vi "Main.vi"() -> ()   [LabVIEW 2015]
uses:
  State.ctl
  Power Meter/Parent/Power Meter.lvclass
  Temperature Device/Parent/Temperature Device.lvclass
  Global Data.ctl
  Data.ctl
  Power Meter/Parent/Power Data.ctl
  <vilib>/Utility/config.llb/Read Key (I32).vi
  <vilib>/Utility/config.llb/Read Key (Double).vi
  <vilib>/Utility/config.llb/Read Key (String).vi
  <vilib>/Utility/config.llb/NI_LVConfig.lvlib
panel:
  out "Channel 3":dbl(graph)
  in  "Simulate":bool
  out "GPIB Error":errorcluster
  out "current time":timestamp format="%<%H:%M:%S%2u>T"
  out "Temperature":cluster{"Data[0]":dbl, "Data[1]":dbl}(graph)
  in  "disp":T1(ring) caption="Display Variable"
  out "Channel 2":dbl(graph)
  out "Channel 1":dbl(graph)
  in  "texe":i32=100
  in  "twait":dbl=1.0
  # "Actual"
  # "Simulated"
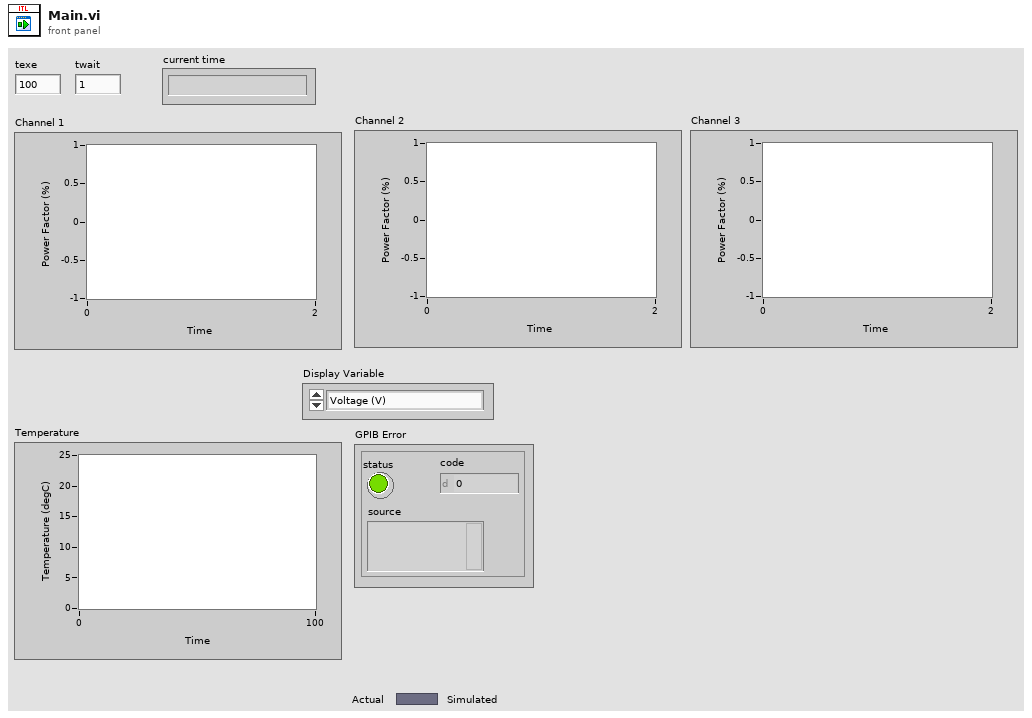
[diagram p1: front panel]
types:
  T1 = enum16{"Voltage (V)", "Amperage (A)", "Power (W)", "Power Factor (%)", "Total Voltage Distortion (%)", "Total Amperage Distortion (%)"}
  T2 = typedef "State.ctl" = enum16{"Configure", "Collect Data", "Wait", "Stop"}
  T3 = typedef "Global Data.ctl" = cluster{"Power Data":T4[], "Time":timestamp, "Temperature":dbl[]}
  T4 = typedef "Data.ctl" = cluster{"Voltage":dbl, "Amperage":dbl, "Wattage":dbl, "Power Factor":dbl, "Voltage Distortion":dbl, "Amperage Distortion":dbl}
  T5 = typedef "Power Meter.lvclass/Power Data.ctl" = cluster{"V":dbl, "I":dbl, "P":dbl, "PF":dbl, "VTHD":dbl, "ITHD":dbl}
  T6 = typedef "NI_LVConfig.lvlib/Config Data RefNum.ctl" = refnum<k1>
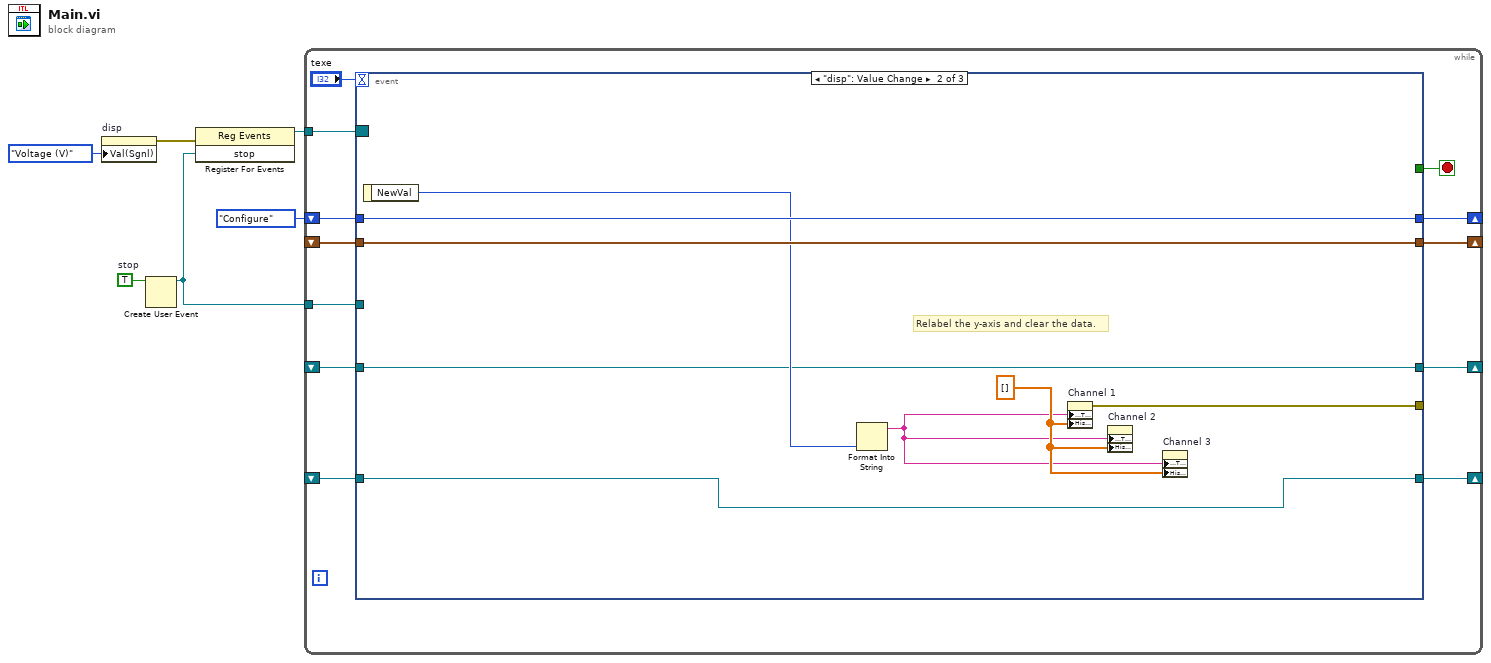
[diagram p0: block diagram]
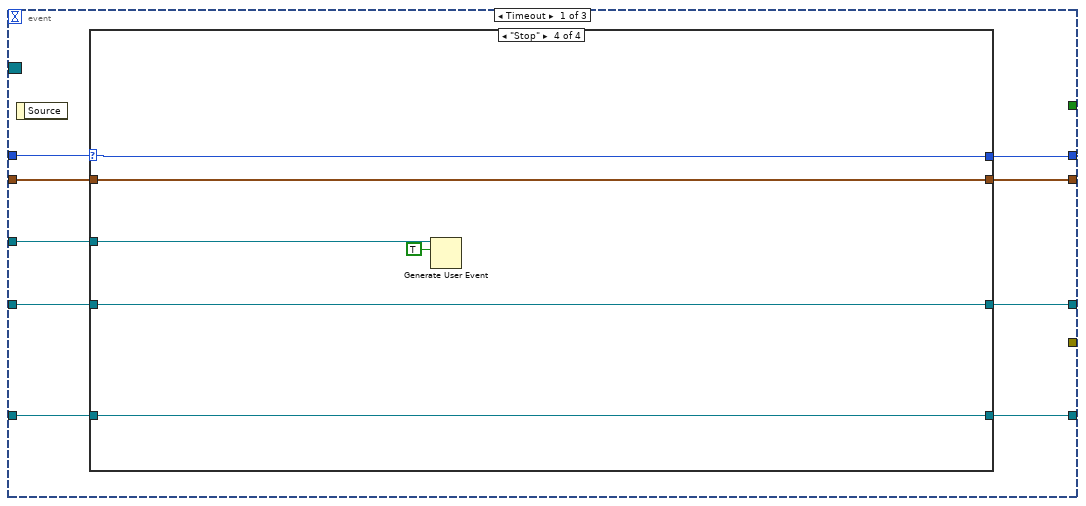
[diagram p2: hidden frame]
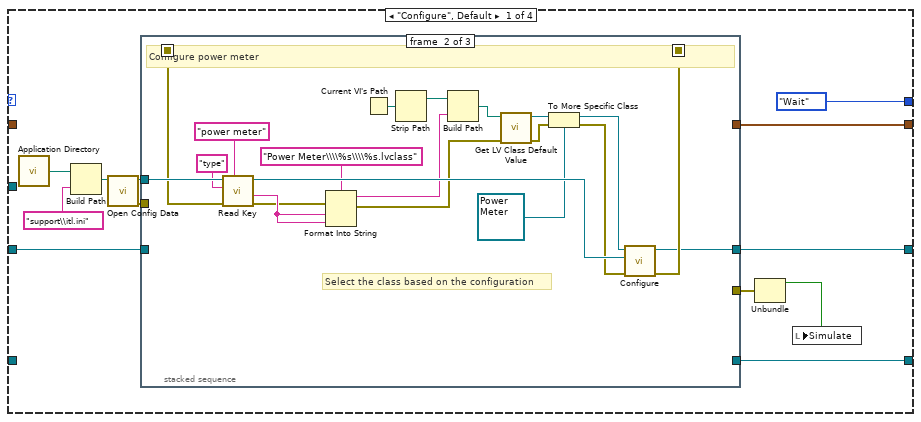
[diagram p3: hidden frame]
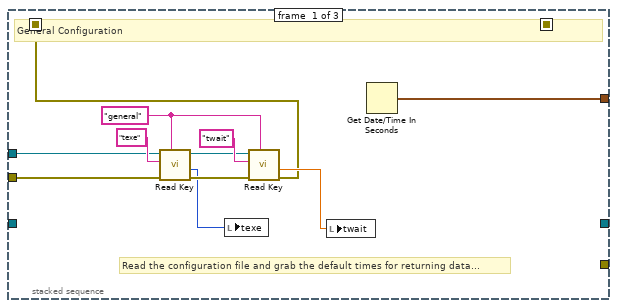
[diagram p4: hidden frame]
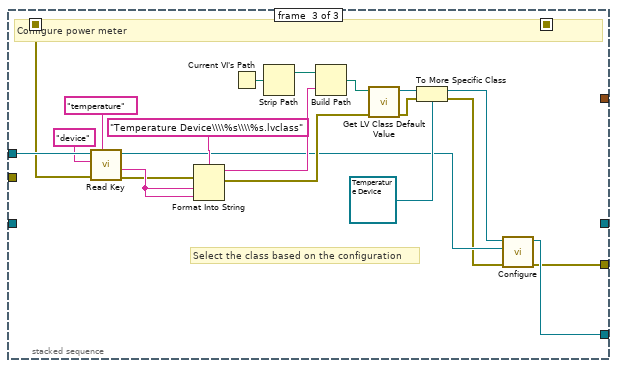
[diagram p5: hidden frame]
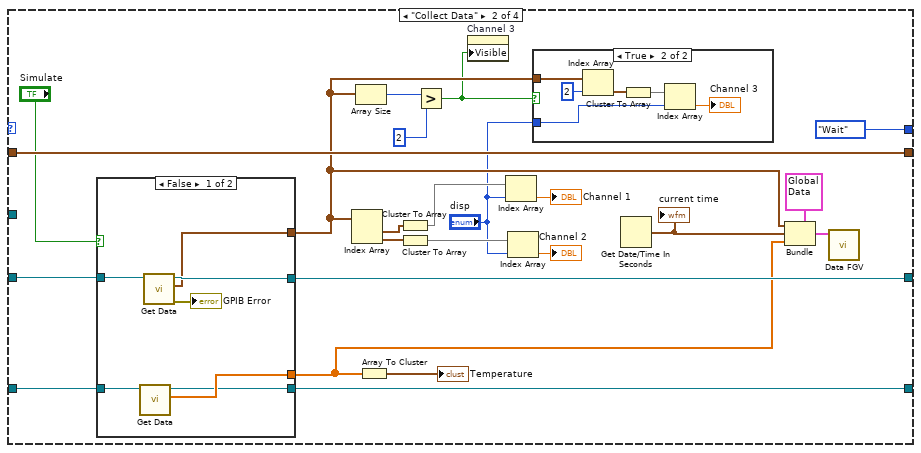
[diagram p6: hidden frame]
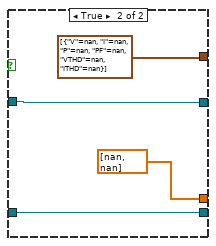
[diagram p8: hidden frame]
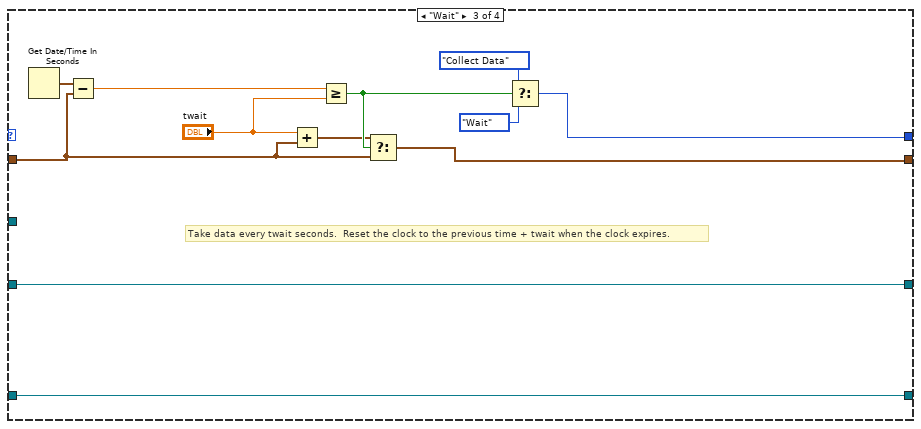
[diagram p9: hidden frame]
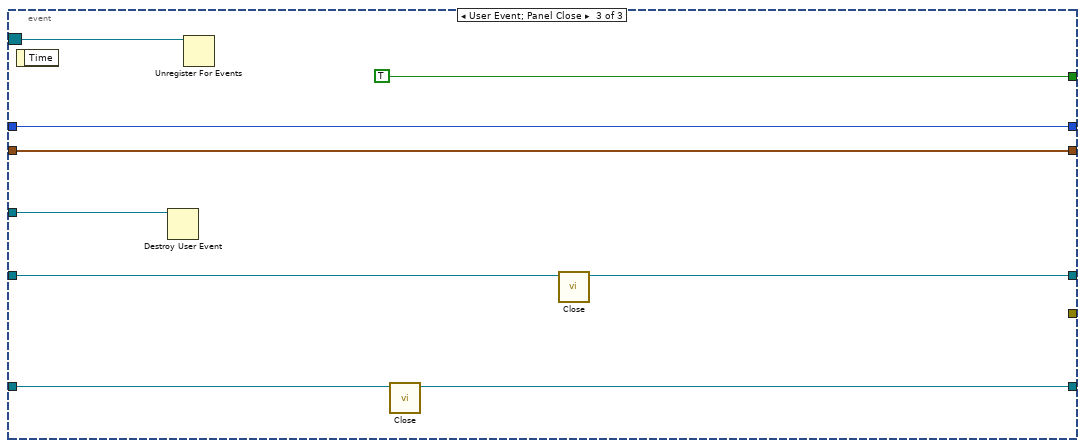
[diagram p10: hidden frame]
diagram:
  w5 = TRUE  # stop
  n1 = property on="disp" class="Enum (strict)"("Val(Sgnl)"=T1."Voltage (V)" ("Value (Signaling)")) -> (error out=w1:errorcluster)  [unwired: 2 in, 1 out]
  n2 = Create User Event(user event datatype=w5) -> (user event=w3:refnum<user-event>)  [unwired: 1 in, 1 out]
  n3 = register-events(error in=w1, w3) -> (reference out=w4:refnum<event-registration>)  [unwired: 1 in, 1 out]
  n4 = while {
    shift-right: [w14] -> _
    shift-left: _ -> [w16]
    shift-right: [w17] -> _
    shift-left: State."Configure" -> [w18]
    tunnel: w4 -> [w13]
    tunnel: w3 -> [w12]
    shift-right: [w9] -> _
    shift-left: _ -> [w10]
    shift-right: [w8] -> _
    shift-left: _ -> [w7]
    stop <- w15 stop-if-true
    n5 = event shown="[1] \"disp\": Value Change" {
      selector: w13 -> [_ _ w161]
      dyn-events: _ -> [_ _ _]
      timeout: "texe" -> [_ _ _]
      tunnel: w18 -> [w27 w155 w163]
      tunnel: [w26 w155 w163] -> w17
      tunnel: w16 -> [w25 w156 w164]
      tunnel: [_ _ TRUE] -> w15
      tunnel: [w24 w156 w164] -> w14
      tunnel: [_ w154 _] -> _
      tunnel: w12 -> [w23 _ w162]
      tunnel: w10 -> [w22 w152 w160]
      tunnel: [w21 w152 w159] -> w9
      tunnel: [w20 w151 w157] -> w8
      tunnel: w7 -> [w19 w151 w158]
      event Timeout {
        n6 = event-data() -> ()  [unwired: 1 in, 1 out]
        n7 = case shown="\"Stop\"" w27 {
          selector: w27 -> [_ _ _ w146]
          tunnel: [State."Wait" State."Wait" w139 w146] -> w26
          tunnel: w25 -> [_ w112 w134 w145]
          tunnel: [w35 w112 w133 w145] -> w24
          tunnel: w23 -> [_ _ _ w148]
          tunnel: w22 -> [w30 w105 w132 w144]
          tunnel: [w29 w104 w132 w144] -> w21
          tunnel: [w28 w98 w131 w143] -> w20
          tunnel: w19 -> [_ w99 w131 w143]
          frame "Configure", Default {
            n8 = call <vilib>:"Application Directory.vi"() -> ("Application Directory"=w39:path)
            n9 = Build Path(base path=w39, name or relative path="support\\itl.ini") -> (appended path=w37:path)
            n10 = call <vilib>:"Open Config Data.vi"("configuration file path"=w37) -> ("error out"=w34:errorcluster, "refnum"=w36:T6)  [unwired: 8 in, 1 out]
            n11 = stacked-sequence {
              seq-local: [w41 _ _] -> [_ w54 w72]
              seq-local: [_ w70 _] -> [_ _ _]
              tunnel: w36 -> [w45 w68 w90]
              tunnel: [w42 _ _] -> w35
              tunnel: [_ _ w71] -> w33
              tunnel: w34 -> [w40 _ _]
              tunnel: w30 -> [_ _ _]
              tunnel: [_ w69 _] -> w29
              tunnel: [_ _ w73] -> w28
              frame #0 {
                w47 = "general" ("section")
                # "Read the configuration file and grab the default times for returning data..."
                # "General Configuration"
                n12 = call-poly <vilib>:"Read Key.vi"("section"=w47, "error in (no error)"=w40, "key"="texe", "refnum"=w45) -> ("error out"=w50:errorcluster, "value"=w44:i32, "refnum out"=w46:T6)  [unwired: 4 in, 1 out]
                n13 = local write "texe"(w44) -> ()
                n14 = call-poly <vilib>:"Read Key.vi"("section"=w47, "error in (no error)"=w50, "key"="twait", "refnum"=w46) -> ("error out"=w41:errorcluster, "value"=w43:dbl)  [unwired: 4 in, 2 out]
                n15 = local write "twait"(w43) -> ()
                n16 = Get Date/Time In Seconds() -> (seconds since 1Jan1904=w42:timestamp)
              }
              frame #1 {
                # "Select the class based on the configuration"
                # "Configure power meter"
                n17 = call-poly <vilib>:"Read Key.vi"("section"="power meter", "error in (no error)"=w54, "key"="type", "refnum"=w68) -> ("error out"=w53:errorcluster, "value"=w61:string, "refnum out"=w65:T6)  [unwired: 4 in, 1 out]
                n18 = Format Into String(format string="Power Meter\\\\%s\\\\%s.lvclass", error in=w53, w61, w61) -> (resulting string=w60:string, error out=w52:errorcluster)  [unwired: 1 in]
                n19 = Current VI's Path() -> (path=w64:path)
                n20 = Strip Path(path=w64) -> (stripped path=w63:path)  [unwired: 1 out]
                n21 = Build Path(base path=w63, name or relative path=w60) -> (appended path=w59:path)
                n22 = call <vilib>:"Get LV Class Default Value.vi"("error in (no error)"=w52, "class path"=w59) -> ("error out"=w58:errorcluster, "object"=w57:refnum<class>)  [unwired: 8 in]
                n23 = To More Specific Class(target class=refnum<class "Power Meter.lvclass"> refnum ("Power Meter"), reference=w57, error in=w58) -> (specific class reference=w55:refnum<class "Power Meter.lvclass">, error out=w51:errorcluster)
                n24 = call-dynamic "Configure.vi"("error in (no error)"=w51, "ConfigRef In"=w65, "Power Meter in"=w55) -> ("error out"=w70:errorcluster, "Power Meter out"=w69:refnum<class "Power Meter.lvclass">)  [unwired: 7 in]
              }
              frame #2 {
                # "Select the class based on the configuration"
                # "Configure power meter"
                n25 = call-poly <vilib>:"Read Key.vi"("section"="temperature", "error in (no error)"=w72, "key"="device", "refnum"=w90) -> ("error out"=w79:errorcluster, "value"=w84:string, "refnum out"=w75:T6)  [unwired: 4 in, 1 out]
                n26 = Format Into String(format string="Temperature Device\\\\%s\\\\%s.lvclass", error in=w79, w84, w84) -> (resulting string=w83:string, error out=w78:errorcluster)  [unwired: 1 in]
                n27 = Current VI's Path() -> (path=w87:path)
                n28 = Strip Path(path=w87) -> (stripped path=w86:path)  [unwired: 1 out]
                n29 = Build Path(base path=w86, name or relative path=w83) -> (appended path=w82:path)
                n30 = call <vilib>:"Get LV Class Default Value.vi"("error in (no error)"=w78, "class path"=w82) -> ("error out"=w81:errorcluster, "object"=w80:refnum<class>)  [unwired: 8 in]
                n31 = To More Specific Class(target class=refnum<class "Temperature Device.lvclass"> refnum ("Temperature Device"), reference=w80, error in=w81) -> (specific class reference=w76:refnum<class "Temperature Device.lvclass">, error out=w74:errorcluster)
                n32 = call-dynamic "Configure.vi"("error in (no error)"=w74, "ConfigRef In"=w75, "Temperature Device in"=w76) -> ("error out"=w71:errorcluster, "Temperature Device out"=w73:refnum<class "Temperature Device.lvclass">)  [unwired: 7 in]
              }
            }
            n33 = Unbundle(w33) -> ("status"=w32:bool)  [unwired: 2 out]
            n34 = local write "Simulate"(w32) -> ()
          }
          frame "Collect Data" {
            n35 = case shown="False" "Simulate" {
              tunnel: [w122 dbl[] [nan, nan] ("Data")] -> w97
              tunnel: w105 -> [w126 w130]
              tunnel: [w125 w130] -> w104
              tunnel: [w124 T5[] [{"V"=nan, "I"=nan, "P"=nan, "PF"=nan, "VTHD"=nan, "ITHD"=nan}] ("Data Out")] -> w93
              tunnel: w99 -> [w123 w128]
              tunnel: [w121 w128] -> w98
              frame False {
                n36 = call-dynamic "Get Data.vi"("Temperature Device in"=w123) -> ("Data"=w122:dbl[], "Temperature Device out"=w121:refnum<class "Temperature Device.lvclass">)  [unwired: 8 in, 1 out]
                n37 = call-dynamic "Get Data.vi"("Power Meter in"=w126) -> ("error out"=→"GPIB Error":errorcluster, "Data Out"=w124:T5[], "Power Meter out"=w125:refnum<class "Power Meter.lvclass">)  [unwired: 8 in]
              }
              frame True {
              }
            }
            n38 = Index Array(array=w93) -> (element #1=w103:T5, element #2=w101:T5)  [unwired: 2 in]
            n39 = Array Size(array=w93) -> (size(s)=w95:i32)
            n40 = Array To Cluster(array=w97) -> (cluster=→"Temperature":cluster{"Data[0]":dbl, "Data[1]":dbl})
            n41 = Cluster To Array(cluster=w103) -> (array=w102:dbl[])
            n42 = Cluster To Array(cluster=w101) -> (array=w100:dbl[])
            n43 = Greater?(x=w95, y=2) -> (0:w91:bool)
            n44 = property on="Channel 3" class="WFChart (strict)"("Visible"=w91) -> ()  [unwired: 2 in, 2 out]
            n45 = Index Array(array=w102, index="disp") -> (element=→"Channel 1":dbl)
            n46 = Index Array(array=w100, index="disp") -> (element=→"Channel 2":dbl)
            n47 = case shown="True" w91 {
              tunnel: w93 -> [_ w119]
              tunnel: "disp" -> [_ w115]
              frame False {
              }
              frame True {
                n48 = Index Array(array=w119, index=2) -> (element=w117:T5)
                n49 = Cluster To Array(cluster=w117) -> (array=w116:dbl[])
                n50 = Index Array(array=w116, index=w115) -> (element=→"Channel 3":dbl)
              }
            }
            n51 = Get Date/Time In Seconds() -> (seconds since 1Jan1904=w110:timestamp)
            "current time" <- w110
            n52 = Bundle(cluster=T3 {"Power Data"=[], "Time"=timestamp(0 s since 1904-01-01), "Temperature"=[]} ("Data In"), "Power Data"=w93, "Time"=w110, "Temperature"=w97) -> (w109:T3)
            n53 = call "Data FGV.vi"("Data In"=w109) -> ()  [unwired: 10 in, 1 out]
          }
          frame "Wait" {
            # "Take data every twait seconds.  Reset the clock to the previous time + twait when the clock expires."
            n54 = Get Date/Time In Seconds() -> (seconds since 1Jan1904=w142:timestamp)
            n55 = Subtract(x=w142, y=w134) -> (x-y=w141:dbl)
            n56 = Add(x="twait", y=w134) -> (x+y=w135:timestamp)
            n57 = Greater Or Equal?(x=w141, y="twait") -> (x >= y?=w136:bool)
            n58 = Select(t=w135, s=w136, f=w134) -> (s? t:f=w133:timestamp)
            n59 = Select(t=State."Collect Data", s=w136, f=State."Wait") -> (s? t:f=w139:T2)
          }
          frame "Stop" {
            n60 = Generate User Event(user event=w148, event data cluster=TRUE ("event data")) -> ()  [unwired: 2 in, 2 out]
          }
        }
      }
      event "disp": Value Change {
        w150 = dbl[] [] ("History Data")
        # "Relabel the y-axis and clear the data."
        n61 = event-data() -> ("NewVal"=w153:T1)  [unwired: 1 in]
        n62 = Format Into String(w153) -> (resulting string=w149:string)  [unwired: 3 in, 1 out]
        n63 = property on="Channel 1" class="WFChart (strict)"("YScale.NameLbl.Text"=w149, "History Data"=w150) -> (error out=w154:errorcluster)  [unwired: 2 in, 1 out]
        n64 = property on="Channel 2" class="WFChart (strict)"("YScale.NameLbl.Text"=w149, "History Data"=w150) -> ()  [unwired: 2 in, 2 out]
        n65 = property on="Channel 3" class="WFChart (strict)"("YScale.NameLbl.Text"=w149, "History Data"=w150) -> ()  [unwired: 2 in, 2 out]
      }
      event User Event; Panel Close {
        n66 = event-data() -> ()  [unwired: 1 in, 1 out]
        n67 = Destroy User Event(user event=w162) -> ()  [unwired: 1 in, 1 out]
        n68 = Unregister For Events(event registration refnum=w161) -> ()  [unwired: 1 in, 1 out]
        n69 = call-dynamic "Close.vi"("Temperature Device in"=w158) -> ("Temperature Device out"=w157:refnum<class "Temperature Device.lvclass">)  [unwired: 9 in, 1 out]
        n70 = call-dynamic "Close.vi"("Power Meter in"=w160) -> ("Power Meter out"=w159:refnum<class "Power Meter.lvclass">)  [unwired: 9 in, 1 out]
      }
    }
  }
